vi "Get ni_servicemanagement_v1_StopServiceRequest.vi"(8 "error in (no error)":errorcluster, 11 "gRPCid":T2) -> (0 "error out":errorcluster, 2 "package_templatemessage":T1, 3 "gRPCid out":T2)   [LabVIEW 2020, in "LineRegulation.lvlib"]
uses:
  LineRegulation.lvlib
  a51dd2a7-b5c1-4c09-9df4-8cd9d3bd0c19.vi
  ni_servicemanagement_v1_StopServiceRequest.ctl
  <vilib>/gRPC/LabVIEW gRPC Library/Server API/typeDefs/grpcId.ctl
  <vilib>/gRPC/LabVIEW gRPC Library/gprc-lvsupport-release.lvlib
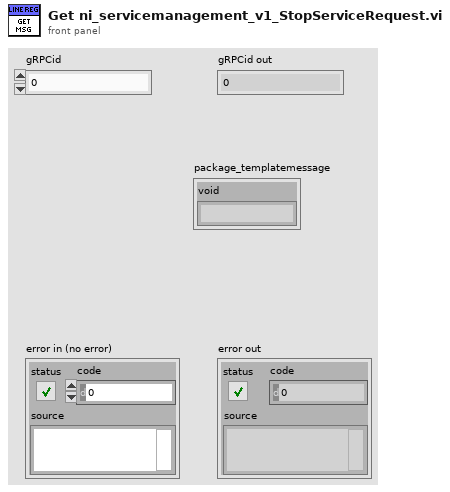
[diagram p1: front panel]
types:
  T1 = typedef "LineRegulation.lvlib/ni_servicemanagement_v1_StopServiceRequest.ctl" = cluster{"void":string}
  T2 = typedef "gprc-lvsupport-release.lvlib/grpcId.ctl" = u64
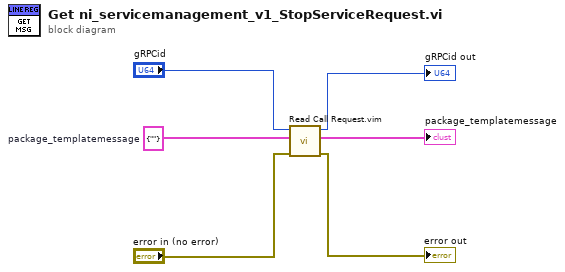
[diagram p0: block diagram]
diagram:
  w2 = T1 {"void"=""}  # package_templatemessage
  n1 = call "Read Call Request.vim"("error in (no error)"="error in (no error)", "Data Type"=w2, "gRPCid in"="gRPCid") -> ("error out"=→"error out":errorcluster, "Request Data"=→"package_templatemessage":T1, "gRPCid out"=→"gRPCid out":T2)  [unwired: 6 in]
